vi "Zadanie_01.vi"() -> ()   [LabVIEW 2020]
uses:
  #typedef_Database.ctl
  <vilib>/Utility/miscctls.llb/LVPositionTypeDef.ctl
panel:
  out "To be moved":dbl
  in  "Sound intensity: MAX":dbl
  in  "Sound intensity: MIN":dbl
  out "Limit exceeded?":bool
  in  "STOP":bool
  in  "Sound intensity [dB]":u8(slide) scale=-7.0..91.0
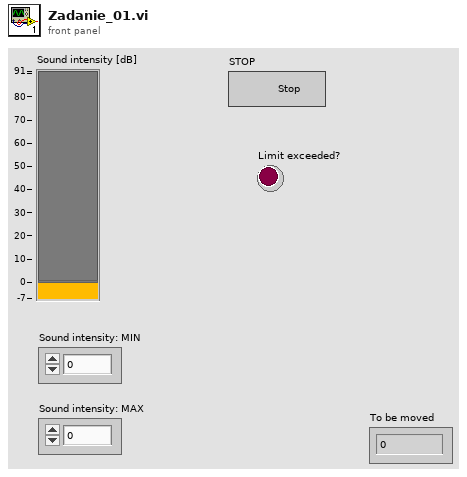
[diagram p1: front panel]
types:
  T1 = typedef "#typedef_Database.ctl" = cluster{"Letters":i16[], "Moving":bool}
  T2 = typedef "LVPositionTypeDef.ctl" = cluster{"Left":i32, "Top":i32}
  T3 = typedef "LVPoint32TypeDef.ctl" = cluster{"Horizontal":i32, "Vertical":i32}
  T4 = typedef "LVBoundsTypeDef.ctl" = cluster{"Width":u32, "Height":u32}
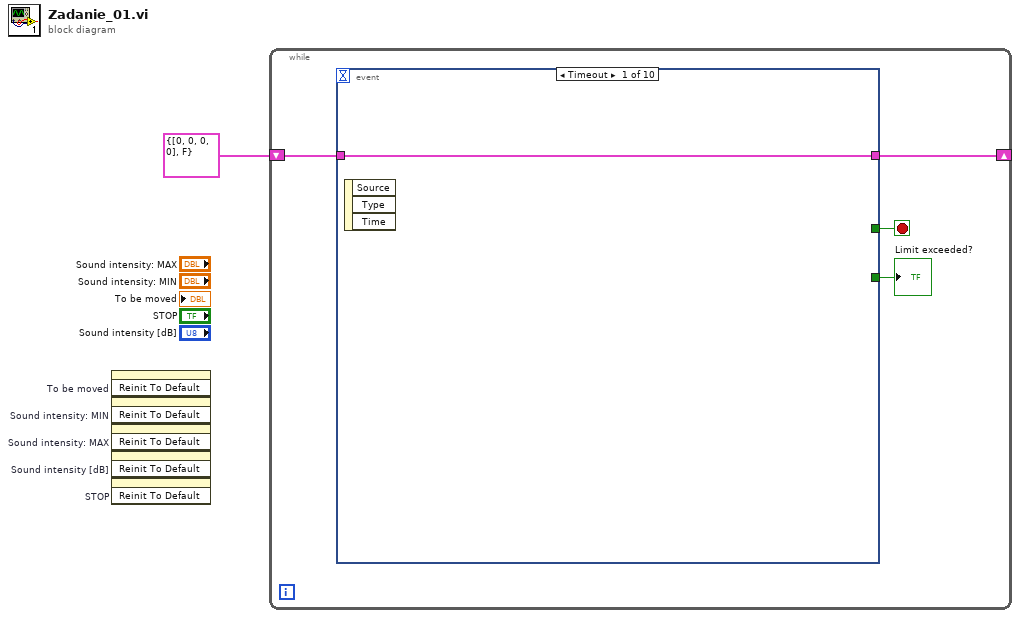
[diagram p0: block diagram]
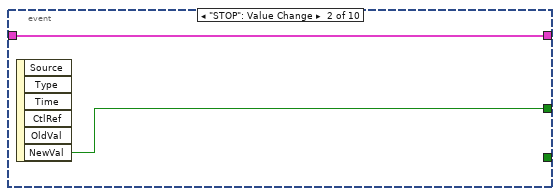
[diagram p2: hidden frame]
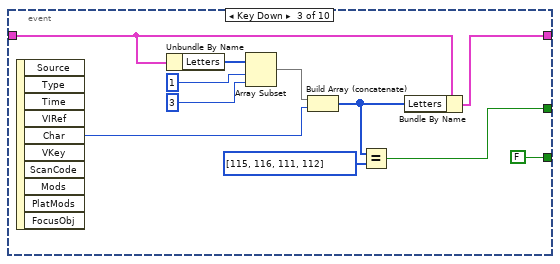
[diagram p3: hidden frame]
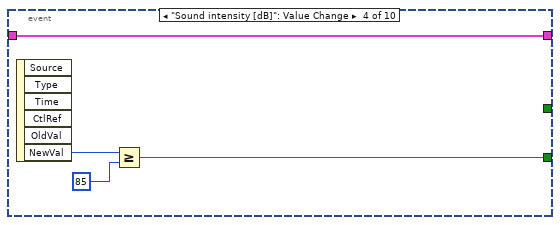
[diagram p4: hidden frame]
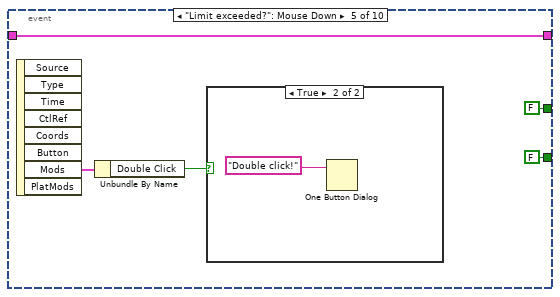
[diagram p5: hidden frame]
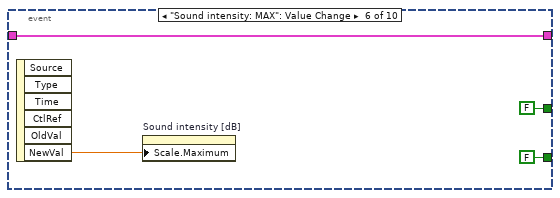
[diagram p7: hidden frame]
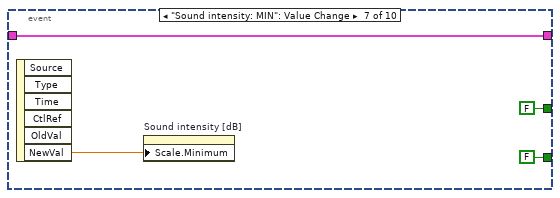
[diagram p8: hidden frame]
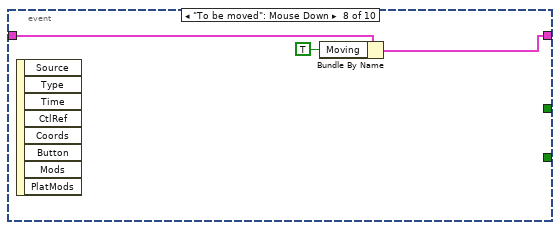
[diagram p9: hidden frame]
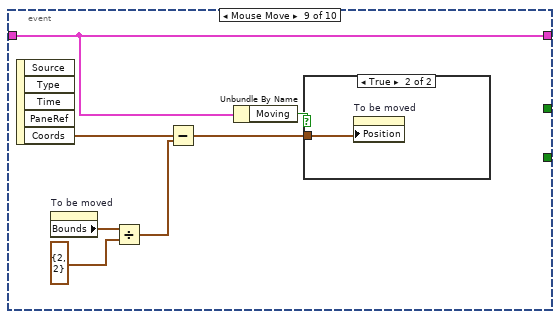
[diagram p10: hidden frame]
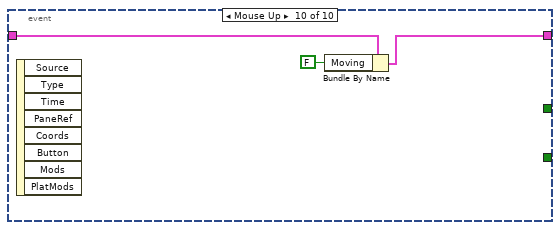
[diagram p12: hidden frame]
diagram:
  n1 = invoke on="To be moved" class="DigNum (strict)" method="Reinit To Default"() -> ()  [unwired: 3 in, 3 out]
  n2 = invoke on="Sound intensity: MIN" class="DigNum (strict)" method="Reinit To Default"() -> ()  [unwired: 3 in, 3 out]
  n3 = invoke on="Sound intensity: MAX" class="DigNum (strict)" method="Reinit To Default"() -> ()  [unwired: 3 in, 3 out]
  n4 = invoke on="Sound intensity [dB]" class="Slide (strict)" method="Reinit To Default"() -> ()  [unwired: 3 in, 3 out]
  n5 = invoke on="STOP" class="Bool" method="Reinit To Default"() -> ()  [unwired: 3 in, 3 out]
  n6 = while {
    shift-right: [w2] -> _
    shift-left: T1 {"Letters"=[0, 0, 0, 0], "Moving"=FALSE} ("Database") -> [w4]
    stop <- w5 stop-if-true
    n7 = event shown="[0] Timeout" {
      selector: _ -> [_ _ _ _ _ _ _ _ _ _]
      dyn-events: _ -> [_ _ _ _ _ _ _ _ _ _]
      timeout: _ -> [_ _ _ _ _ _ _ _ _ _]
      tunnel: [_ w8 w10 _ FALSE ("NewVal") FALSE ("NewVal") FALSE ("NewVal") _ _ _] -> w5
      tunnel: w4 -> [w6 w7 w14 w20 w24 w30 w34 w40 w46 w50]
      tunnel: [w6 w7 w13 w20 w24 w30 w34 w39 w46 w49] -> w2
      tunnel: [_ _ FALSE w21 FALSE FALSE FALSE _ _ _] -> w3
      event Timeout {
        n8 = event-data() -> ()  [unwired: 1 in, 3 out]
      }
      event "STOP": Value Change {
        n9 = event-data() -> ("NewVal"=w8:bool)  [unwired: 1 in, 5 out]
      }
      event Key Down {
        n10 = event-data() -> ("Char"=w15:i16)  [unwired: 1 in, 9 out]
        n11 = Unbundle By Name(w14) -> ("Letters"=w19:i16[])
        n12 = Array Subset(array=w19, index=1, length=3) -> (w16:i16[])
        n13 = Build Array (concatenate)(w16, w15) -> (w12:i16[])
        n14 = Equal?(x=w12, y=i16[] [115, 116, 111, 112]) -> (x = y?=w10:bool)
        n15 = Bundle By Name(cluster=w14, "Letters"=w12) -> (w13:T1)
      }
      event "Sound intensity [dB]": Value Change {
        n16 = event-data() -> ("NewVal"=w23:u8)  [unwired: 1 in, 5 out]
        n17 = Greater Or Equal?(x=w23, y=u8 85) -> (x >= y?=w21:bool)
      }
      event "Limit exceeded?": Mouse Down {
        n18 = event-data() -> ("Mods"=w28:cluster{"Double Click":bool, "Menu Key":bool})  [unwired: 1 in, 7 out]
        n19 = Unbundle By Name(w28) -> ("Double Click"=w27:bool)
        n20 = case shown="True" w27 {
          frame False {
          }
          frame True {
            n21 = One Button Dialog(message="Double click!") -> ()  [unwired: 1 in, 1 out]
          }
        }
      }
      event "Sound intensity: MAX": Value Change {
        n22 = event-data() -> ("NewVal"=w33:dbl)  [unwired: 1 in, 5 out]
        n23 = property on="Sound intensity [dB]" class="Slide (strict)"("Scale.Maximum"=w33) -> ()  [unwired: 2 in, 2 out]
      }
      event "Sound intensity: MIN": Value Change {
        n24 = event-data() -> ("NewVal"=w37:dbl)  [unwired: 1 in, 5 out]
        n25 = property on="Sound intensity [dB]" class="Slide (strict)"("Scale.Minimum"=w37) -> ()  [unwired: 2 in, 2 out]
      }
      event "To be moved": Mouse Down {
        n26 = event-data() -> ()  [unwired: 1 in, 8 out]
        n27 = Bundle By Name(cluster=w40, "Moving"=TRUE) -> (w39:T1)
      }
      event Mouse Move {
        n28 = event-data() -> ("Coords"=w43:T3)  [unwired: 1 in, 4 out]
        n29 = property on="To be moved" class="DigNum (strict)"() -> ("Bounds"=w45:T4)  [unwired: 2 in, 2 out]
        n30 = Divide(x=w45, y=T2 {"Left"=2, "Top"=2}) -> (x/y=w42:cluster{dbl, dbl})
        n31 = Subtract(x=w43, y=w42) -> (x-y=w41:cluster{dbl, dbl})
        n32 = Unbundle By Name(w46) -> ("Moving"=w47:bool)
        n33 = case shown="True" w47 {
          tunnel: w41 -> [_ w48]
          frame False {
          }
          frame True {
            n34 = property on="To be moved" class="DigNum (strict)"("Position"=w48) -> ()  [unwired: 2 in, 2 out]
          }
        }
      }
      event Mouse Up {
        n35 = event-data() -> ()  [unwired: 1 in, 8 out]
        n36 = Bundle By Name(cluster=w50, "Moving"=FALSE) -> (w49:T1)
      }
    }
    "Limit exceeded?" <- w3
  }
